vi "Read BMP File (excel).vi"(8 "error in (no error)":errorcluster, 11 "path to BMP file":path) -> (0 "error out":errorcluster, 1 "flattened image data":u8[](array[numeric]), 2 "rect":T1, 3 "path":path, 4 "color table":u32[](array[colorbox]), 5 "depth":u8)   [LabVIEW 2017, in "NI_ReportGenerationToolkit.lvlib"]
doc: "Reads a Windows bitmap file and creates the data necessary for the file to be displayed in a Picture control."
uses:
  <vilib>/addons/_office/NI_ReportGenerationToolkit.lvlib
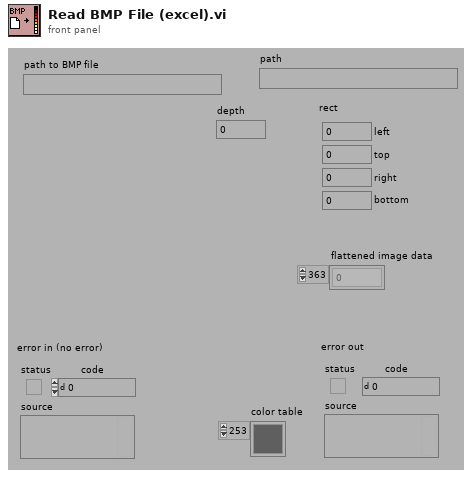
[diagram p1: front panel]
types:
  T1 = cluster{"left":i16, "top":i16, "right":i16, "bottom":i16}
  T2 = cluster{"height":u32, "width":u32, "bit depth":u16, "padded width":u32}
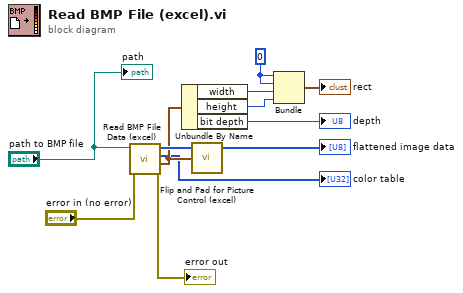
[diagram p0: block diagram]
diagram:
  w10 = i16 0
  n1 = call <vilib>:"Read BMP File Data (excel).vi"("error in (no error)"="error in (no error)", "path to BMP file"="path to BMP file") -> ("error out"=→"error out":errorcluster, "bitmap info"=w11:T2, "color table"=→"color table":u32[], "BMP data"=w12:u8[])  [unwired: 6 out]
  n2 = Unbundle By Name(w11) -> ("width"=w9:u32, "height"=w8:u32, "bit depth"=→"depth":u16)
  n3 = call <vilib>:"Flip and Pad for Picture Control (excel).vi"("bitmap info"=w11, "BMP bitmap"=w12) -> ("picture bitmap"=→"flattened image data":u8[])  [unwired: 1 in, 2 out]
  n4 = Bundle(w10, w10, "width"=w9, "height"=w8) -> (→"rect":cluster{i16, i16, "width":u32, "height":u32})  [unwired: 1 out]
  "path" <- "path to BMP file"
